vi "prueba_botones.vi"() -> ()   [LabVIEW 2019]
panel:
  in  "2":dbl caption="Posición final en Y"
  in  "1":dbl caption="Posición final en X"
  in  "stop":bool
  in  "Motores independientes":bool
  out "String":string
  in  "Trayectoria":bool
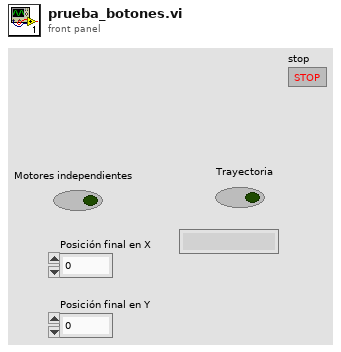
[diagram p1: front panel]
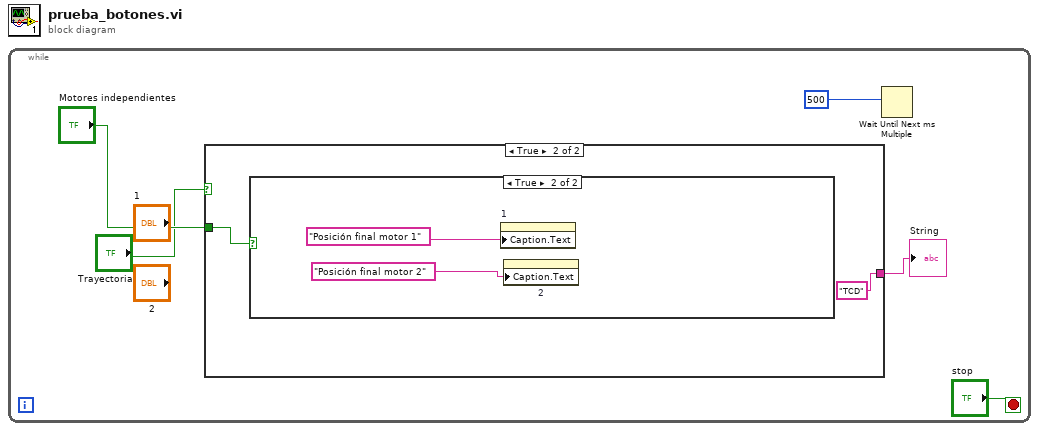
[diagram p0: block diagram]
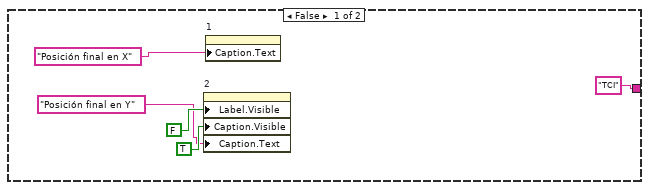
[diagram p2: hidden frame]
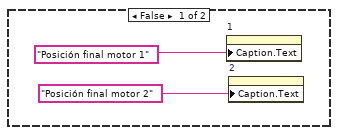
[diagram p3: hidden frame]
diagram:
  n1 = while {
    stop <- "stop" stop-if-true
    n2 = case shown="True" "Trayectoria" {
      tunnel: ["TCI" "TCD"] -> w5
      tunnel: "Motores independientes" -> [_ w11]
      frame False {
        n3 = property on="2" class="DigNum (strict)"("Label.Visible"=FALSE, "Caption.Visible"=TRUE, "Caption.Text"="Posición final en Y") -> ()  [unwired: 2 in, 2 out]
        n4 = property on="1" class="DigNum (strict)"("Caption.Text"="Posición final en X") -> ()  [unwired: 2 in, 2 out]
      }
      frame True {
        n5 = case shown="True" w11 {
          frame False {
            n6 = property on="1" class="DigNum (strict)"("Caption.Text"="Posición final motor 1") -> ()  [unwired: 2 in, 2 out]
            n7 = property on="2" class="DigNum (strict)"("Caption.Text"="Posición final motor 2") -> ()  [unwired: 2 in, 2 out]
          }
          frame True {
            n8 = property on="1" class="DigNum (strict)"("Caption.Text"="Posición final motor 1") -> ()  [unwired: 2 in, 2 out]
            n9 = property on="2" class="DigNum (strict)"("Caption.Text"="Posición final motor 2") -> ()  [unwired: 2 in, 2 out]
          }
        }
      }
    }
    "String" <- w5
    n10 = Wait Until Next ms Multiple(millisecond multiple=500) -> ()  [unwired: 1 out]
  }
